vi "Read General Setting from PVM.vi"(11 "UI General Setting in":T1) -> (3 "UI General Setting out":T1)   [LabVIEW 2015, in "ConfigHelper.lvlib"]
uses:
  ConfigHelper.lvlib
  Control_UI_General Setting.ctl
  Control_UI_General Setting State.ctl
  <vilib>/addons/PointValueMap/controls/PointMap.ctl
  <vilib>/addons/PointValueMap/PointValueMap.lvlib
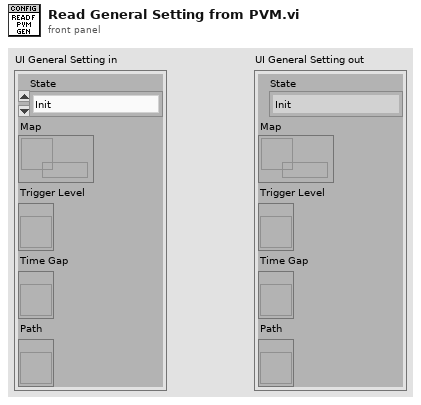
[diagram p1: front panel]
types:
  T1 = typedef "ConfigHelper.lvlib/Control_UI_General Setting.ctl" = cluster{"State":T2, "Map":T3, "Trigger Level":refnum<vi>, "Time Gap":refnum<vi>, "Path":refnum<vi>}
  T2 = typedef "ConfigHelper.lvlib/Control_UI_General Setting State.ctl" = enum16{"Init", "Read from PVM", "Wait", "Write to PVM", "Exit"}
  T3 = typedef "PointValueMap.lvlib/PointMap.ctl" = refnum<data-value>
  T4 = typedef "ConfigHelper.lvlib/Control_General Setup (Path).ctl" = cluster{"Export Path":path, "level":dbl, "Time Gap":dbl}
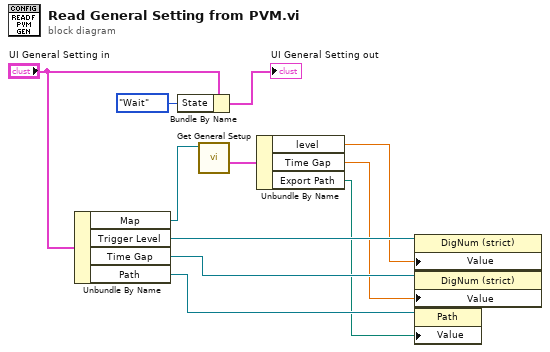
[diagram p0: block diagram]
diagram:
  n1 = Unbundle By Name("UI General Setting in") -> ("Map"=w5:T3, "Trigger Level"=w11:refnum<vi>, "Time Gap"=w10:refnum<vi>, "Path"=w9:refnum<vi>)
  n2 = Bundle By Name(cluster="UI General Setting in", "State"=Control_UI_General_Setting_State."Wait") -> (→"UI General Setting out":T1)
  n3 = call "Get General Setup.vi"("Map"=w5) -> ("General Setup"=w4:T4)  [unwired: 8 in, 2 out]
  n4 = Unbundle By Name(w4) -> ("level"=w1:dbl, "Time Gap"=w2:dbl, "Export Path"=w3:path)
  n5 = property class="DigNum (strict)"(reference=w11, "Value"=w1) -> ()  [unwired: 1 in, 2 out]
  n6 = property class="DigNum (strict)"(reference=w10, "Value"=w2) -> ()  [unwired: 1 in, 2 out]
  n7 = property class="Path"(reference=w9, "Value"=w3) -> ()  [unwired: 1 in, 2 out]
